vi "SET - Triggered Events & Data.vi"(8 "error in (no error)":errorcluster, 9 "Data":string="Hi!!!", 10 "Events":T1, 11 "Child_2_Class in":refnum<class "Console_Class.lvclass">) -> (0 "error out":errorcluster, 3 "Child_2_Class out":refnum<class "Console_Class.lvclass">)   [LabVIEW 2023, in "Console_Actor.lvlib" / "Console_Class.lvclass"]
uses:
  Console_Class.lvclass
  Abstraction_Interface_Class/Usr Ev/Ctrl - Enum - Events.ctl
  Console_Class.lvclass/Console_Class.ctl
  Abstraction_Interface_Class/Abstraction_Interface_Class.lvclass
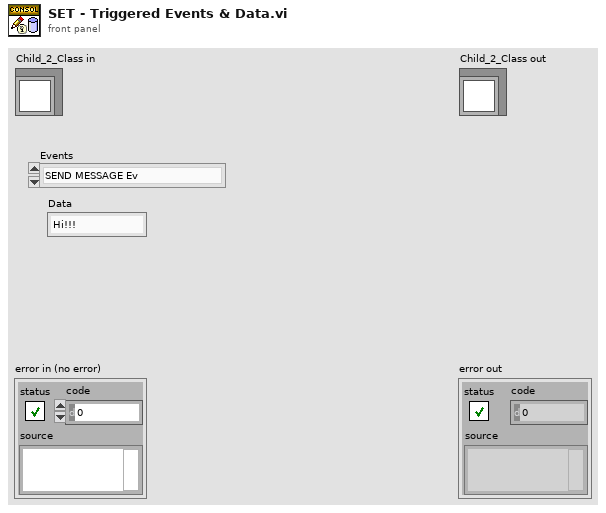
[diagram p1: front panel]
types:
  T1 = typedef "Abstraction_Interface.lvlib/Abstraction_Interface_Class.lvclass/Ctrl - Enum - Events.ctl" = enum16{"SEND MESSAGE Ev", "STOP_ACTOR Ev", "INIT_ACTOR Ev", "START Ev", "STOP Ev", "GET Ev", "SET Ev", "ERROR_HANDLER Ev", "RESET Ev"}
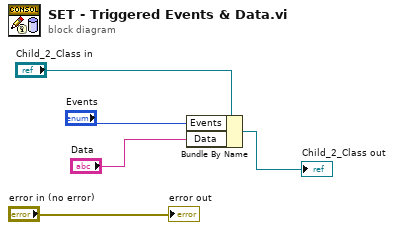
[diagram p0: block diagram]
diagram:
  n1 = Bundle By Name(cluster="Child_2_Class in", "Events"="Events", "Data"="Data") -> (→"Child_2_Class out":refnum<class "Console_Class.lvclass">)
  "error out" <- "error in (no error)"
